vi "CoefficientOverlays.vi"(6 "plotInfoArray":T2(array[cluster]), 7 "\"At\" location":T4={"XcoordSys"="graph", "YcoordSys"="graph", "Xvalue"=0.05, "Yvalue"=0.92}, 9 "BL Targets":T1[](array[typedef]) {"n" min=0.02 max=0.5 step=0.01 format="%.2f"}, 10 "Coefficients":cluster{"No d0":T3, "with d0":T3}, 11 "gnuplotIn":string) -> (3 "gnuplotOut":string)   [LabVIEW 2014]
uses:
  at.ctl
  PowerLaw.ctl
  BLTarget.ctl
panel:
  out "resulting string":string
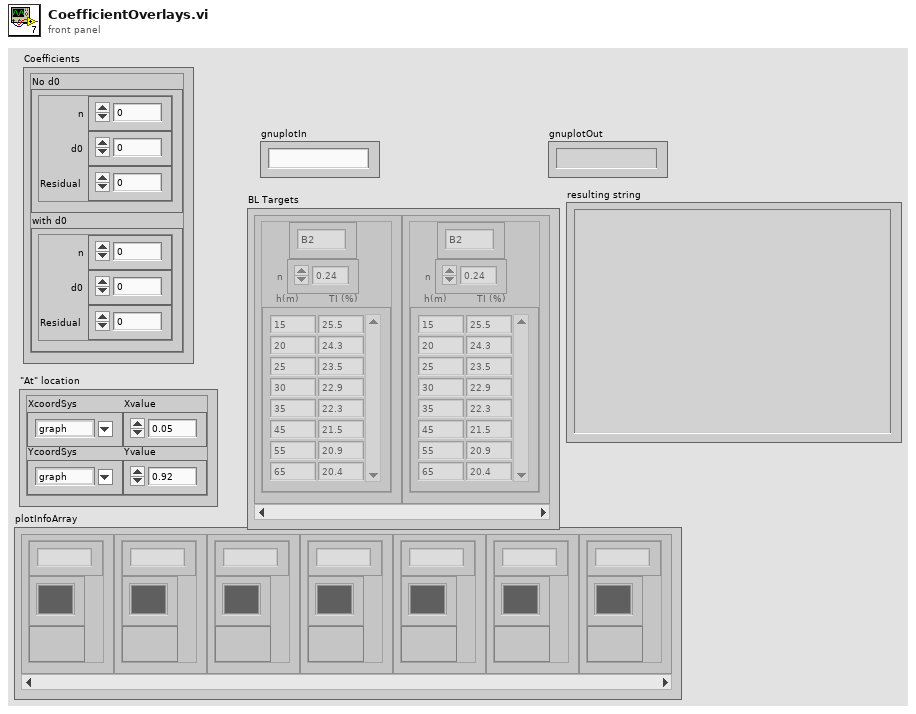
[diagram p1: front panel]
types:
  T1 = typedef "BLTarget.ctl" = cluster{"Code":string, "TI Profile (FS)":dbl[][], "n":dbl}
  T2 = cluster{"Plot Name":string, "Plot.Plot Color":u32, "Plot.Visible?":bool}[]
  T3 = typedef "PowerLaw.ctl" = cluster{"n":dbl, "d0":dbl, "Residual":dbl}
  T4 = typedef "at.ctl" = cluster{"XcoordSys":string, "YcoordSys":string, "Xvalue":dbl, "Yvalue":dbl}
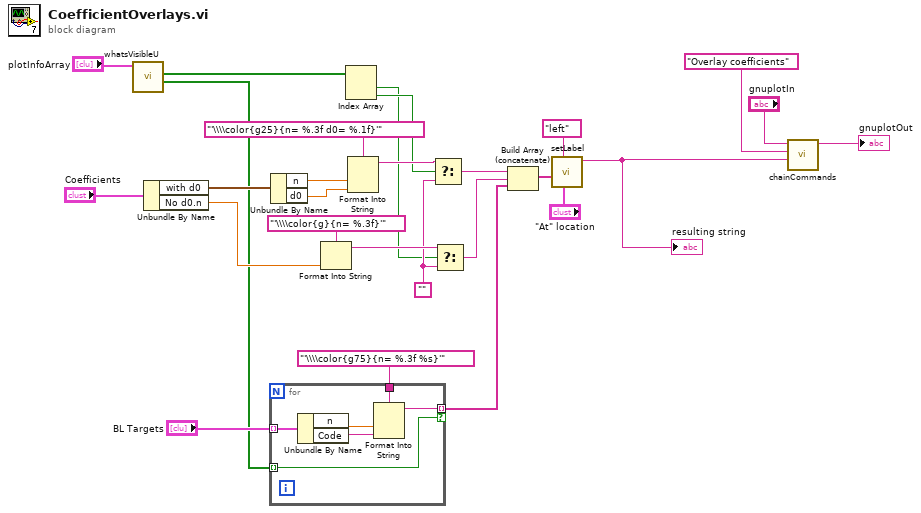
[diagram p0: block diagram]
diagram:
  w13 = ""
  n1 = call "whatsVisibleU.vi"("UplotInfoArray"="plotInfoArray") -> ("Targets Visible"=w4:bool[], "Fits Visible"=w1:bool[])  [unwired: 8 in, 1 out]
  n2 = Unbundle By Name("Coefficients") -> ("with d0"=w19:T3, "No d0.n"=w18:dbl)
  n3 = for {
    tunnel: "'\\\\color{g75}{n= %.3f %s}'" ("format string") -> [w33]
    tunnel: [w32] -> w6 mode=indexing if=w28
    tunnel: w4 -> [w28] mode=indexing
    tunnel: "BL Targets" -> [w31] mode=indexing
    n4 = Unbundle By Name(w31) -> ("n"=w30:dbl, "Code"=w29:string)
    n5 = Format Into String(format string=w33, w30, w29) -> (resulting string=w32:string)  [unwired: 2 in, 1 out]
  }
  n6 = Unbundle By Name(w19) -> ("n"=w27:dbl, "d0"=w25:dbl)
  n7 = Format Into String(format string="'\\\\color{g}{n= %.3f}'", w18) -> (resulting string=w16:string)  [unwired: 2 in, 1 out]
  n8 = Index Array(array=w1) -> (element #1=w2:bool, element #2=w3:bool)  [unwired: 2 in]
  n9 = Format Into String(format string="'\\\\color{g25}{n= %.3f d0= %.1f}'", w27, w25) -> (resulting string=w17:string)  [unwired: 2 in, 1 out]
  n10 = Select(t=w17, s=w3, f=w13) -> (s? t:f=w15:string)
  n11 = Select(t=w16, s=w2, f=w13) -> (s? t:f=w14:string)
  n12 = Build Array (concatenate)(w15, w14, w6) -> (w21:string[])
  n13 = call "setLabel.vi"("\"At\" location"="\"At\" location", "Justify"="left", "multilineLabel"=w21) -> ("String out"=w12:string)  [unwired: 7 in, 1 out]
  "resulting string" <- w12
  n14 = call "chainCommands.vi"("Command"=w12, "Comments"="Overlay coefficients", "StringIn"="gnuplotIn") -> ("StringOut"=→"gnuplotOut":string)  [unwired: 8 in]
